vi "Handle.vi"(11 "Base Queue Actor in":refnum<class "Base Queue Actor.lvclass">) -> (2 "Destroy?":bool, 3 "Base Queue Actor out":refnum<class "Base Queue Actor.lvclass">)   [LabVIEW 2021, in "jettl.lvlib" / "Base Queue Actor.lvclass"]
uses:
  Base Queue Actor.lvclass
  C:/git/jettl/src/jettl/Queue Actor/Queue Actor.lvclass
  Base Queue Actor.lvclass/Base Queue Actor.ctl
  Queue State/Queue State/Queue State.lvclass
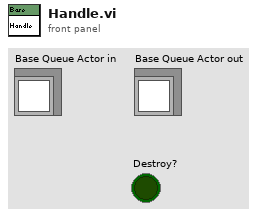
[diagram p1: front panel]
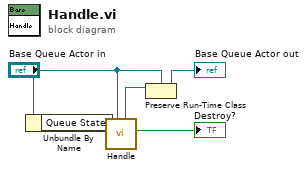
[diagram p0: block diagram]
diagram:
  n1 = Unbundle By Name("Base Queue Actor in") -> ("Queue State"=w5:refnum<class "Queue State.lvclass">)
  n2 = call-dynamic "Handle.vi"("Queue Actor in"="Base Queue Actor in", "Queue State in"=w5) -> ("Destroy?"=→"Destroy?":bool, "Queue Actor out"=w4:refnum<class "Queue Actor.lvclass">)  [unwired: 8 in]
  n3 = Preserve Run-Time Class(object in=w4, 2:"Base Queue Actor in") -> (object out=→"Base Queue Actor out":refnum<class "Base Queue Actor.lvclass">)  [unwired: 1 in, 1 out]
